vi "Append Chapter bookmark.vi"(0 "PDF Report":refnum<class "PDF Report Class.lvclass">, 1 "Chapter or section":T1, 2 "Title":string, 3 "Title indentation":T2, 5 "TriggerNewPage (Chapter)":bool=TRUE, 11 "error in (no error)":errorcluster, 12 "Font":T6={"Name"="", "Size"=-1.0, "Color"=0, "Style"={"Bold"=TRUE, "Italic"=FALSE, "Underline"=FALSE, "Strikeout"=FALSE}, "Type"={"Type&direction"=enum."Select", "Embedded"=FALSE, "Encoding"=""}}, 14 "Title properties":T3={" Aligment"=enum."LEFT", "Line spacing"=enum."Select"}) -> (4 "PDF Report duplicate":refnum<class "PDF Report Class.lvclass">, 15 "error out":errorcluster)   [LabVIEW 2019, in "Exaprom PDF.lvlib"]
doc: "<B>Only ASCII or UTF-16 (no-bidi).</B>\n\nAppends text with a <B>line feed</B>, at the end, to the PDF report. This text can be <B>aligned</B> (CENTER, JUSTIFY, LEFT, RIGHT) and <B>indented</B>. \n\nIf <B>Font</B> and <B>Pararaph properties</B> are not specified then the <B>Default font</B> and <B>Default paragraph</B> will be use.\n\nThe data type you wire to the <B>Text</B> input determines the polymorphic instance to use.\n\n<B>FRANÇAIS</B>\nAjoute au rapport PDF du texte sous la forme d'un paragraphe terminé avec un \"<B>Line Feed</B>\". Ce texte peut être <B>aligné</B> (CENTER, JUSTIFY, LEFT, RIGHT) et avoir un <B>renfoncement</B> (gauche et droit) pour tout le paragraphe.\n\nSi la police de caractères <B>Font</B> et les propriétés <B>Pararaph properties</B> ne sont pas spécifiés alors la police par défaut <B>Default font</B> et <B>Default paragraph</B> seront utilisées.\n\nLe type de données que vous connectez au terminal <B>Text</B> détermine l'instance polymorphique utilisée.\n\nVersion 2.0\nDeveloped by Jean-Marc Simard\nCopyright © 2013, Exaprom Inc.\nAll rights reserved.\nLicense: BSD\n\nWith iTextSharp 4.1.6 (http://itextsharp.sourceforge.net)\nunder Mozilla Public License Version 1.1\n(http://www.mozilla.org/MPL/MPL-1.1.html)"
uses:
  Controls/Font Controls/Font complete cluster.ctl
  Controls/Font Controls/Font size.ctl
  Controls/Font Controls/Font color.ctl
  Controls/Font Controls/Type and encoding.ctl
  Controls/Text Controls/Unicode/Type and run direction.ctl
  Controls/Initialization Controls/Defaut Paragraphe and Line Spacing.ctl
  Controls/Text Controls/Texte alignement.ctl
  Controls/Text Controls/Line spacing.ctl
  LV Class/PDF Report Class/PDF Report Class.lvclass
  Controls/Text Controls/Paragraph indentation.ctl
  Controls/Chapter Controls/Chapter.ctl
  Controls/Text Controls/Phrase or paragraph.ctl
  Controls/Text Controls/Unicode/Source rub direction.ctl
  C:/work/niobrara_lv/labview pdf writer fixing/DLL/itextsharp.dll
  DLL/itextsharp.dll
  Exaprom PDF.lvlib
  LV Class/Fonts Class/Font Class.lvclass
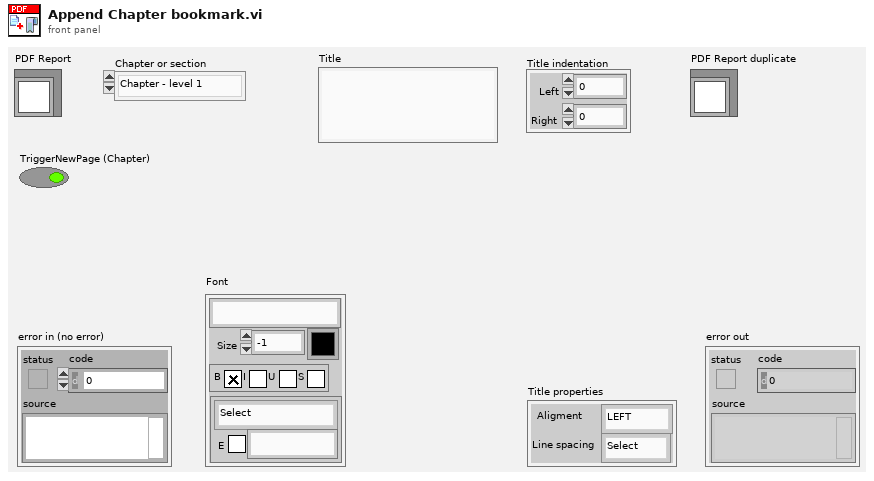
[diagram p1: front panel]
types:
  T1 = typedef "Exaprom PDF.lvlib/Chapter.ctl" = enum16{"Chapter - level 1", "Chapter - level 2", "Chapter - level 3", "Chapter - level 4"}
  T2 = typedef "Exaprom PDF.lvlib/Paragraph indentation.ctl" = cluster{"Left":sgl, "Right":sgl}
  T3 = typedef "Exaprom PDF.lvlib/Defaut Paragraphe and Line Spacing.ctl" = cluster{" Aligment":T4, "Line spacing":T5}
  T4 = typedef "Exaprom PDF.lvlib/Texte alignement.ctl" = enum16{"Select", "CENTER", "JUSTIFY", "LEFT", "RIGHT"}
  T5 = typedef "Exaprom PDF.lvlib/Line spacing.ctl" = enum16{"Select", "1.0", "1.5", "2.0"}
  T6 = typedef "Exaprom PDF.lvlib/Font complete cluster.ctl" = cluster{"Name":string, "Size":T7, "Color":T8, "Style":cluster{"Bold":bool, "Italic":bool, "Underline":bool, "Strikeout":bool}, "Type":T9}
  T7 = typedef "Exaprom PDF.lvlib/Font size.ctl" = sgl
  T8 = typedef "Exaprom PDF.lvlib/Font color.ctl" = u32
  T9 = typedef "Exaprom PDF.lvlib/Type and encoding.ctl" = cluster{"Type&direction":T10, "Embedded":bool, "Encoding":string}
  T10 = typedef "Exaprom PDF.lvlib/Type and run direction.ctl" = enum16{"Select", "ASCII", "UTF-16", "UTF-16 (default)", "UTF-16 (LTR)", "UTF-16 (RTL)"}
  T11 = typedef "Exaprom PDF.lvlib/Source rub direction.ctl" = enum16{"Chapter", "Paragraph", "Phrase", "pdfpcell"}
  T12 = typedef "Exaprom PDF.lvlib/Phrase or paragraph.ctl" = enum16{"Add to Phrase", "Add to Paragraph", "Create Phrase", "Create Paragraph"}
  T13 = typedef "Exaprom PDF.lvlib/Unit.ctl" = enum16{"inch", "mm"}
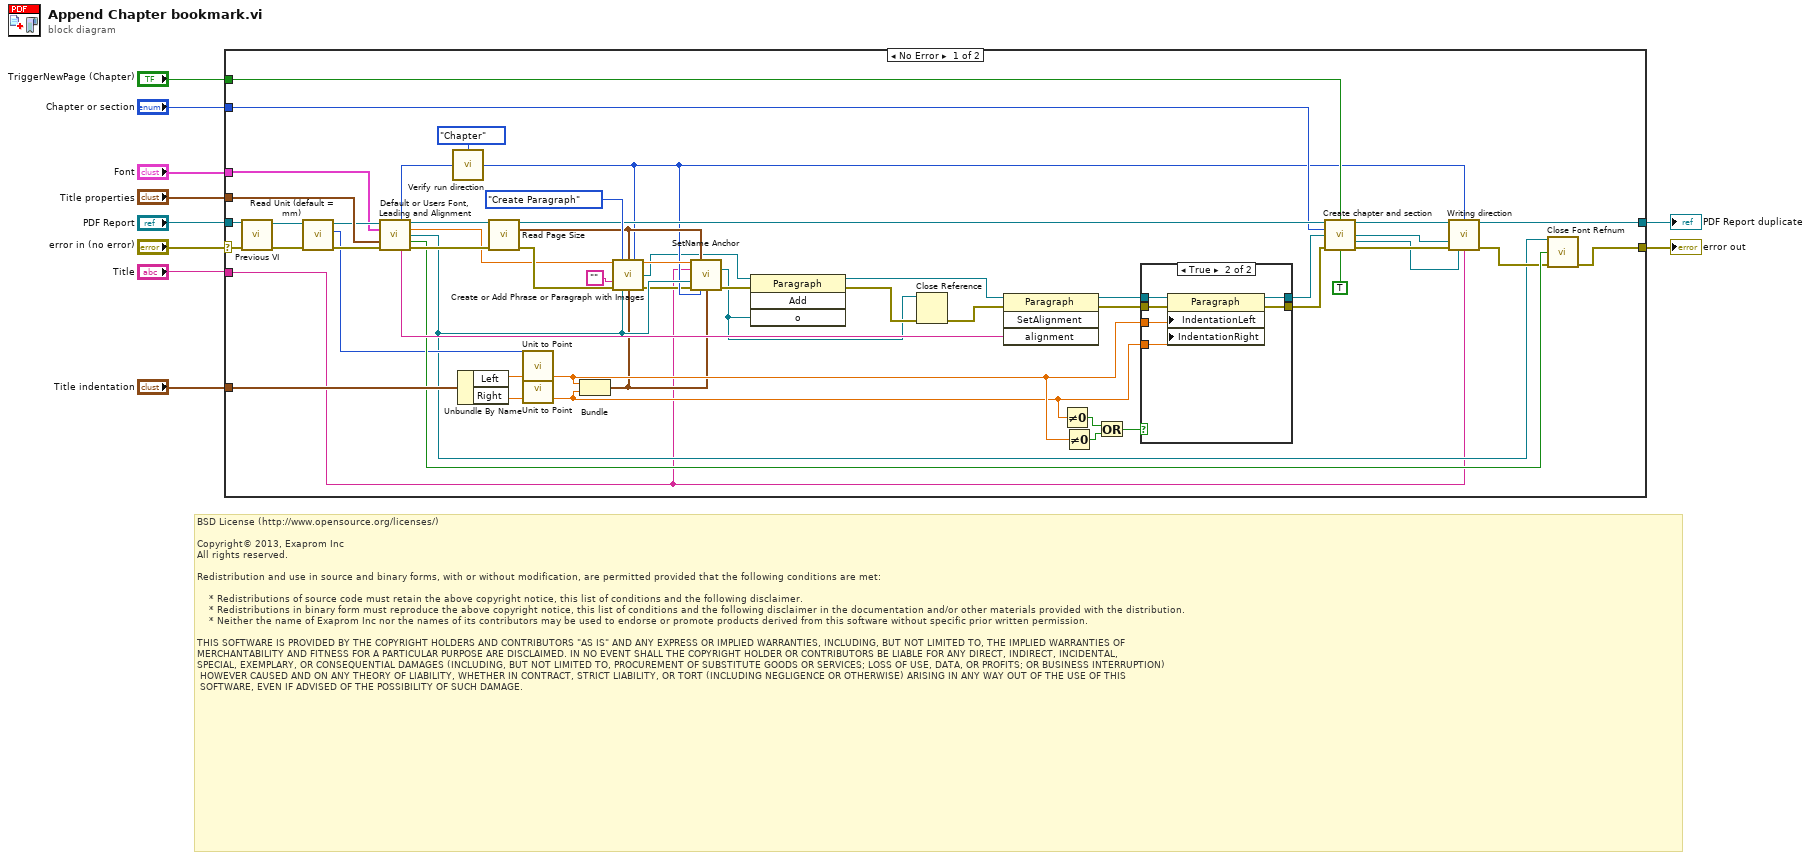
[diagram p0: block diagram]
diagram:
  # "BSD License (http://www.opensource.org/licenses/)\n\nCopyright© 2013, Exaprom Inc\nAll rights reserved.\n\nRedistribution and use in source and binary forms, with or without modification, are permitted provided that the following conditions are met:\n\n    * Redistributions of source code must retain the above copyright notice, this list of conditions and the following disclaimer.\n    * Redistributions in binary form must reproduce the above copyright notice, this list of conditions and the following disclaimer in the documentation and/or other materials provided with the distribution.\n    * Neither the name of Exaprom Inc nor the names of its contributors may be used to endorse or promote products derived from this software without specific prior written permission.\n\nTHIS SOFTWARE IS PROVIDED BY THE COPYRIGHT HOLDERS AND CONTRIBUTORS \"AS IS\" AND ANY EXPRESS OR IMPLIED WARRANTIES, INCLUDING, BUT NOT LIMITED TO, THE IMPLIED WARRANTIES OF \nMERCHANTABILITY AND FITNESS FOR A PARTICULAR PURPOSE ARE DISCLAIMED. IN NO EVENT SHALL THE COPYRIGHT HOLDER OR CONTRIBUTORS BE LIABLE FOR ANY DIRECT, INDIRECT, INCIDENTAL,\nSPECIAL, EXEMPLARY, OR CONSEQUENTIAL DAMAGES (INCLUDING, BUT NOT LIMITED TO, PROCUREMENT OF SUBSTITUTE GOODS OR SERVICES; LOSS OF USE, DATA, OR PROFITS; OR BUSINESS INTERRUPTION)\n HOWEVER CAUSED AND ON ANY THEORY OF LIABILITY, WHETHER IN CONTRACT, STRICT LIABILITY, OR TORT (INCLUDING NEGLIGENCE OR OTHERWISE) ARISING IN ANY WAY OUT OF THE USE OF THIS\n SOFTWARE, EVEN IF ADVISED OF THE POSSIBILITY OF SUCH DAMAGE."
  n1 = case shown="No Error" "error in (no error)" {
    selector: "error in (no error)" -> [w44 w74]
    tunnel: "Font" -> [w30 _]
    tunnel: "Title" -> [w18 _]
    tunnel: [w52 w74] -> w9
    tunnel: "PDF Report" -> [w56 w73]
    tunnel: "Title properties" -> [w55 _]
    tunnel: [w42 w73] -> w5
    tunnel: "Title indentation" -> [w62 _]
    tunnel: "TriggerNewPage (Chapter)" -> [w33 _]
    tunnel: "Chapter or section" -> [w32 _]
    frame No Error {
      n2 = call "Previous VI.vi"("PDF Report IN"=w56, "error in (no error)"=w44) -> ("PDF Report OUT"=w29:refnum<class "PDF Report Class.lvclass">, "error out"=w28:errorcluster)  [unwired: 12 out]
      n3 = call-dynamic "Read Unit (default = mm).vi"("error in (no error)"=w28, "PDF Report Class in"=w29) -> ("error out"=w50:errorcluster, "Unit (default = mm)"=w48:T13, "PDF Report Class out"=w49:refnum<class "PDF Report Class.lvclass">)  [unwired: 7 in]
      n4 = call "Default or Users Font, Leading and Alignment.vi"("PDF Report"=w49, "Font"=w30, "Paragraphe cluster"=w55, "error in (no error)"=w50) -> ("Type and run direction"=w27:T10, "PDF Report duplicate"=w53:refnum<class "PDF Report Class.lvclass">, "Leading"=w23:T7, "Font Ref"=w22:refnum<k24>, "Close Font Ref"=w51:bool, "Aligment"=w64:string, "error out"=w54:errorcluster)  [unwired: 5 out]
      n5 = call "Verify run direction.vi"("Source"=Source_rub_direction."Chapter", "Type&direction IN"=w27) -> ("Type&direction OUT"=w21:T10)  [unwired: 2 in]
      n6 = Unbundle By Name(w62) -> ("Left"=w58:sgl, "Right"=w57:sgl)
      n7 = call "Read Page Size.vi"("PDF Report"=w53, "error in (no error)"=w54) -> ("PDF Report duplicate"=w41:refnum<class "PDF Report Class.lvclass">, "Text zone (points)"=w24:cluster{"widht":sgl, "height":sgl}, "error out"=w39:errorcluster)  [unwired: 11 out]
      n8 = call "Unit to Point.vi"("X unit"=w58, "Unit (default = mm)"=w48) -> ("X point"=w46:sgl)  [unwired: 7 out]
      n9 = call "Unit to Point.vi"("X unit"=w57, "Unit (default = mm)"=w48) -> ("X point"=w45:sgl)  [unwired: 7 out]
      n10 = Bundle("X point"=w46, "X point"=w45) -> (w20:cluster{" X point":sgl, " X point":sgl})  [unwired: 1 out]
      n11 = call "Create or Add Phrase or Paragraph with Images.vi"("Leading"=w23, "Phrase or paragraph"=Phrase_or_paragraph."Create Paragraph", "Text zone (points)"=w24, "Character type"=w21, "Text"="", "error in (no error)"=w39, "Font refnum"=w22, "Paragraph indentation (points)"=w20) -> ("Paragraph refnum OUT"=w12:refnum<k24>, "error out"=w19:errorcluster)  [unwired: 3 in, 3 out]
      n12 = call "SetName Anchor.vi"("Leading"=w23, "Text zone (points)"=w24, "Text"=w18, "Font refnum"=w22, "error in (no error)"=w19, "Type and run direction"=w21, "Paragraph indentation (points)"=w20) -> ("Anchor"=w13:refnum<k24>, "error out"=w17:errorcluster)  [unwired: 6 in, 1 out]
      n13 = invoke class="Paragraph" method="Add"(reference=w12, error in=w17, "o"=w13) -> (reference out=w15:refnum<k24>, error out=w16:errorcluster)  [unwired: 1 in, 2 out]
      n14 = Close Reference(reference=w13, error in (no error)=w16) -> (error out=w14:errorcluster)
      n15 = invoke class="Paragraph" method="SetAlignment"(reference=w15, error in=w14, "alignment"=w64) -> (reference out=w40:refnum<k24>, error out=w63:errorcluster)  [unwired: 1 in, 2 out]
      n16 = Not Equal To 0?(x=w45) -> (x != 0?=w60:bool)
      n17 = Not Equal To 0?(x=w46) -> (x != 0?=w59:bool)
      n18 = Or(x=w60, y=w59) -> (x .or. y?=w61:bool)
      n19 = case shown="True" w61 {
        tunnel: w40 -> [w66 w72]
        tunnel: w63 -> [w65 w71]
        tunnel: [w65 w70] -> w36
        tunnel: [w66 w69] -> w35
        tunnel: w46 -> [_ w68]
        tunnel: w45 -> [_ w67]
        frame False {
        }
        frame True {
          n20 = property class="Paragraph"(reference=w72, error in=w71, "IndentationLeft"=w68, "IndentationRight"=w67) -> (reference out=w69:refnum<k24>, error out=w70:errorcluster)
        }
      }
      n21 = call "Create chapter and section.vi"("PDF Report IN"=w41, "TriggerNewPage"=w33, "Chapter or section IN"=w32, "Paragragh"=w35, "error in (no error)"=w36, "BookmarkOpen"=TRUE) -> ("PDF Report OUT"=w38:refnum<class "PDF Report Class.lvclass">, "Chapter"=w31:refnum<k24>, "Section"=w34:refnum<k24>, "error out"=w37:errorcluster)  [unwired: 6 in]
      n22 = call "Writing direction.vi"("PDF Report IN"=w38, "Text type"=w21, "ChapterAutoNumber"=w31, "error in (no error)"=w37, "Section"=w34, "Title"=w18) -> ("PDF Report OUT"=w42:refnum<class "PDF Report Class.lvclass">, "error out"=w43:errorcluster)  [unwired: 8 in]
      n23 = call "Close Font Refnum.vi"("Font Refnum"=w22, "Close ?"=w51, "error in (no error)"=w43) -> ("error out"=w52:errorcluster)  [unwired: 12 in]
    }
    frame Error {
    }
  }
  "error out" <- w9
  "PDF Report duplicate" <- w5
